vi "PWM.vi"(0 "Refnum in":refnum<k21>, 5 "Speed 1":dbl, 7 "error in (no error)":errorcluster, 10 "High Time In 1":dbl) -> (20 "Refnum out":refnum<k21>, 22 "High Time Out 1":dbl, 27 "error out":errorcluster)   [LabVIEW 2011]
uses:
  <vilib>/DAQmx/write.llb/DAQmx Write (Counter Time 1Chan 1Samp).vi
  <vilib>/DAQmx/miscellaneous.llb/DAQmx Fill In Error Info.vi
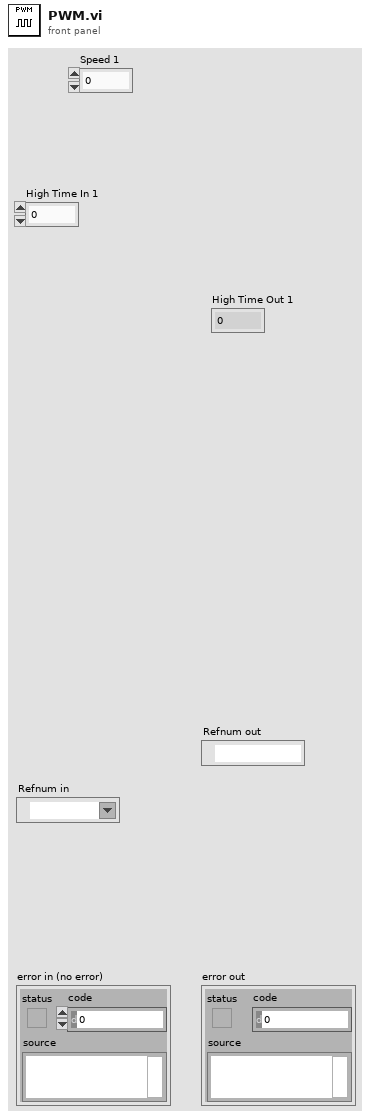
[diagram p1: front panel]
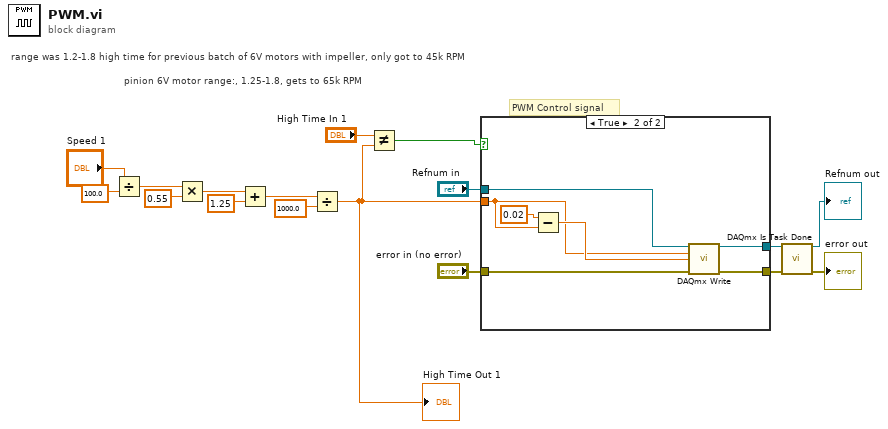
[diagram p0: block diagram]
diagram:
  # "pinion 6V motor range:, 1.25-1.8, gets to 65k RPM"
  # "range was 1.2-1.8 high time for previous batch of 6V motors with impeller, only got to 45k RPM"
  # "PWM Control signal"
  n1 = Divide(x="Speed 1", y=100.0) -> (x/y=w9:dbl)
  n2 = Multiply(x=w9, y=0.55 ("scale")) -> (x*y=w11:dbl)
  n3 = Add(x=w11, y=1.25 ("add")) -> (x+y=w7:dbl)
  n4 = Divide(x=w7, y=1000.0) -> (x/y=w3:dbl)
  "High Time Out 1" <- w3
  n5 = Not Equal?(x="High Time In 1", y=w3) -> (x != y?=w1:bool)
  n6 = case shown="True" w1 {
    tunnel: [w19 w26] -> w15
    tunnel: [w18 w25] -> w16
    tunnel: "Refnum in" -> [w19 w24]
    tunnel: "error in (no error)" -> [w18 w23]
    tunnel: w3 -> [_ w20]
    frame False {
    }
    frame True {
      n7 = Subtract(x=0.02 ("total time"), y=w20) -> (x-y=w21:dbl)
      n8 = call-poly <vilib>:"DAQmx Write.vi"("task/channels in"=w24, "high time"=w20, "low time"=w21, "error in"=w23) -> ("task out"=w26:refnum<k21>, "error out"=w25:errorcluster)  [unwired: 9 in, 1 out]
    }
  }
  n9 = call <vilib>:"DAQmx Is Task Done.vi"("task/channels in"=w15, "error in"=w16) -> ("task out"=→"Refnum out":refnum<k21>, "error out"=→"error out":errorcluster)  [unwired: 11 in, 1 out]
